vi "ExperimentCode.vi"() -> ()   [LabVIEW 2017]
uses:
  <vilib>/Instr/_visa.llb/VISA Configure Serial Port (Instr).vi
  <vilib>/express/express shared/transition.llb/Dynamic To Waveform Array.vi
  <vilib>/express/express signal manip/GetorSetDDTAttributes/Set DDT Attributes/SetT0.vi
  <vilib>/express/express shared/transition.llb/Waveform Array To Dynamic.vi
  <vilib>/express/express signal manip/GetorSetDDTAttributes/Set DDT Attributes/Set DDT Properties.xnode
  <vilib>/Analysis/NI_AALPro.lvlib
panel:
  in  "Yaw Moment Intercept":dbl
  in  "Yaw Moment Slope":dbl
  in  "Lift Force Intercept":dbl
  in  "Lift Force Slope":dbl
  in  "Drag Force Intercept":dbl
  in  "Drag Force Slope":dbl
  in  "Tab Control":enum32{"Setup ", "Experiment Controls", "Debug"}(tab)=enum."Experiment Controls"
  in  "Max Torque":dbl=21.3
  in  "Servo 1 Zero Offset":dbl
  in  "Servo 2 Zero Offset":dbl
  in  "Servo 3 Zero Offset":dbl
  in  "Servo 4 Zero Offset":dbl
  in  "Servo 5 Zero Offset":dbl
  in  "Servo 5 Torque Intercept":dbl=-52.5
  in  "Servo 5 Torque Slope":dbl=0.0021
  in  "Servo 5 Position Intercept":dbl=-125.0
  in  "Servo 5 Position Slope":dbl=0.007
  in  "Servo 4 Torque Intercept":dbl=-52.5
  in  "Servo 4 Torque Slope":dbl=0.0021
  in  "Servo 4 Position Intercept":dbl=-125.0
  in  "Servo 4 Position Slope":dbl=0.007
  in  "Servo 3 Torque Intercept":dbl=-52.5
  in  "Servo 3 Torque Slope":dbl=0.0021
  in  "Servo 3 Position Intercept":dbl=-125.0
  in  "Servo 3 Position Slope":dbl=0.007
  in  "Servo 2 Torque Intercept":dbl=-52.5
  in  "Servo 2 Torque Slope":dbl=0.0021
  in  "Servo 2 Position Intercept":dbl=-125.0
  in  "Servo 2 Position Slope":dbl=0.007
  in  "Servo 1 Torque Intercept":dbl=-52.5
  in  "Servo 1 Torque Slope":dbl=0.0021
  in  "Servo 1 Position Intercept":dbl=-125.0
  in  "Servo 1 Position Slope":dbl=0.007
  in  "Plot Last x Seconds":dbl=5.0
  in  "COM Port":refnum<visa-resource-name>
  in  "Buad Rate":i32(ring)=115200 items=["2400"=2400, "4800"=4800, "9600"=9600, "14400"=14400, "19200"=19200, "28800"=28800, "38400"=38400, "57600"=57600, "115200"=115200]
  in  "Lowest Servo Angle":dbl=15.0
  in  "Highest Servo Angle":dbl=155.0
  out "Lift FFT":cluster{"timeout (s)":dbl, dbl, dbl[]}(graph)
  out "Maximum Torque Exceeded":bool
  in  "Amplitude (deg)":dbl=3.0
  in  "Save":bool
  in  "Stop VI":bool
  in  "Sample Frequency":dbl=10000.0 step=50.0
  out "Servo Torque":cluster{" Time Offset":dbl, dbl, dbl[][]}(graph)
  in  "Amplitude":dbl=4.0
  in  "Length of Segments":dbl=10.0
  in  "Number of Servos":dbl=5.0
  in  "Number of Waves":dbl=1.0
  in  "Wave Exponential":dbl=2.0
  in  "Frequency":dbl=1.0
  in  "Wave Form":u16(ring) items=["Sine", "Exponentional Sine", "Second Mode Bending", "Flat Plate"]
  in  "Wind Up Waveform":bool
  in  "Mode 1 Amplitude":dbl=0.1 step=0.1
  in  "Mode 2 Amplitude":dbl=0.2 step=0.1
  in  "Mode 1 Phase":dbl step=0.1
  in  "Mode 2 Phase":dbl=0.8499 step=0.1
  in  "Wind Down Waveform":bool
  in  "Wind Down Time":i32=5
  out "Waveform":cluster{"X Nodes":dbl[], "Y Nodes":dbl[]}[](graph)
  in  "Servo Input":bool
  in  "Send To Waveform to MBE":bool
  in  "Servo 5 Input":dbl=90.0
  in  "Servo 4 Input":dbl=90.0
  in  "Servo 3 Input":dbl=90.0
  in  "Servo 2 Input":dbl=90.0
  in  "Servo 1 Input":dbl=90.0
  out "Force and Torque Data":cluster{i32, dbl, dbl[][]}(graph)
  out "Minimum or Maximum Angle Exceeded":bool
  in  "Filename":path=path "test.tdms"
  in  "Comment":string
  out "Output Angles":dbl[](array[numeric])
  out "Input Angles":dbl[](array[numeric])
  out "Pos5 number":dbl
  out "Pos4 number":dbl
  out "Pos3 number":dbl
  out "Pos2 number":dbl
  out "Pos1 number":dbl
  out "Torq1 number":dbl
  out "Torq2 number":dbl
  out "Torq3 number":dbl
  out "Torq4 number":dbl
  out "Torq5 number":dbl
  out "Servo 1 Position":cluster{i32, dbl, dbl[][]}(graph)
  out "Servo 2 Position":cluster{i32, dbl, dbl[][]}(graph)
  out "Servo 3 Position":cluster{i32, dbl, dbl[][]}(graph)
  out "Servo 4 Position":cluster{i32, dbl, dbl[][]}(graph)
  out "Servo 5 Position":cluster{i32, dbl, dbl[][]}(graph)
  out "Sent to Arduino":string
  out "Bytes at port":cluster{i32, dbl, dbl[]}(graph)
  out "Read Buffer":string
  # "deg"
  # "deg"
  # "deg"
  # "deg"
  # "deg"
  # "Waveform"
  # "Manual"
  # "cm"
  # "cm"
  # "Hz"
  # "Off"
  # "On"
  # "rad"
  # "rad"
  # "Off"
  # "On"
  # "Hz"
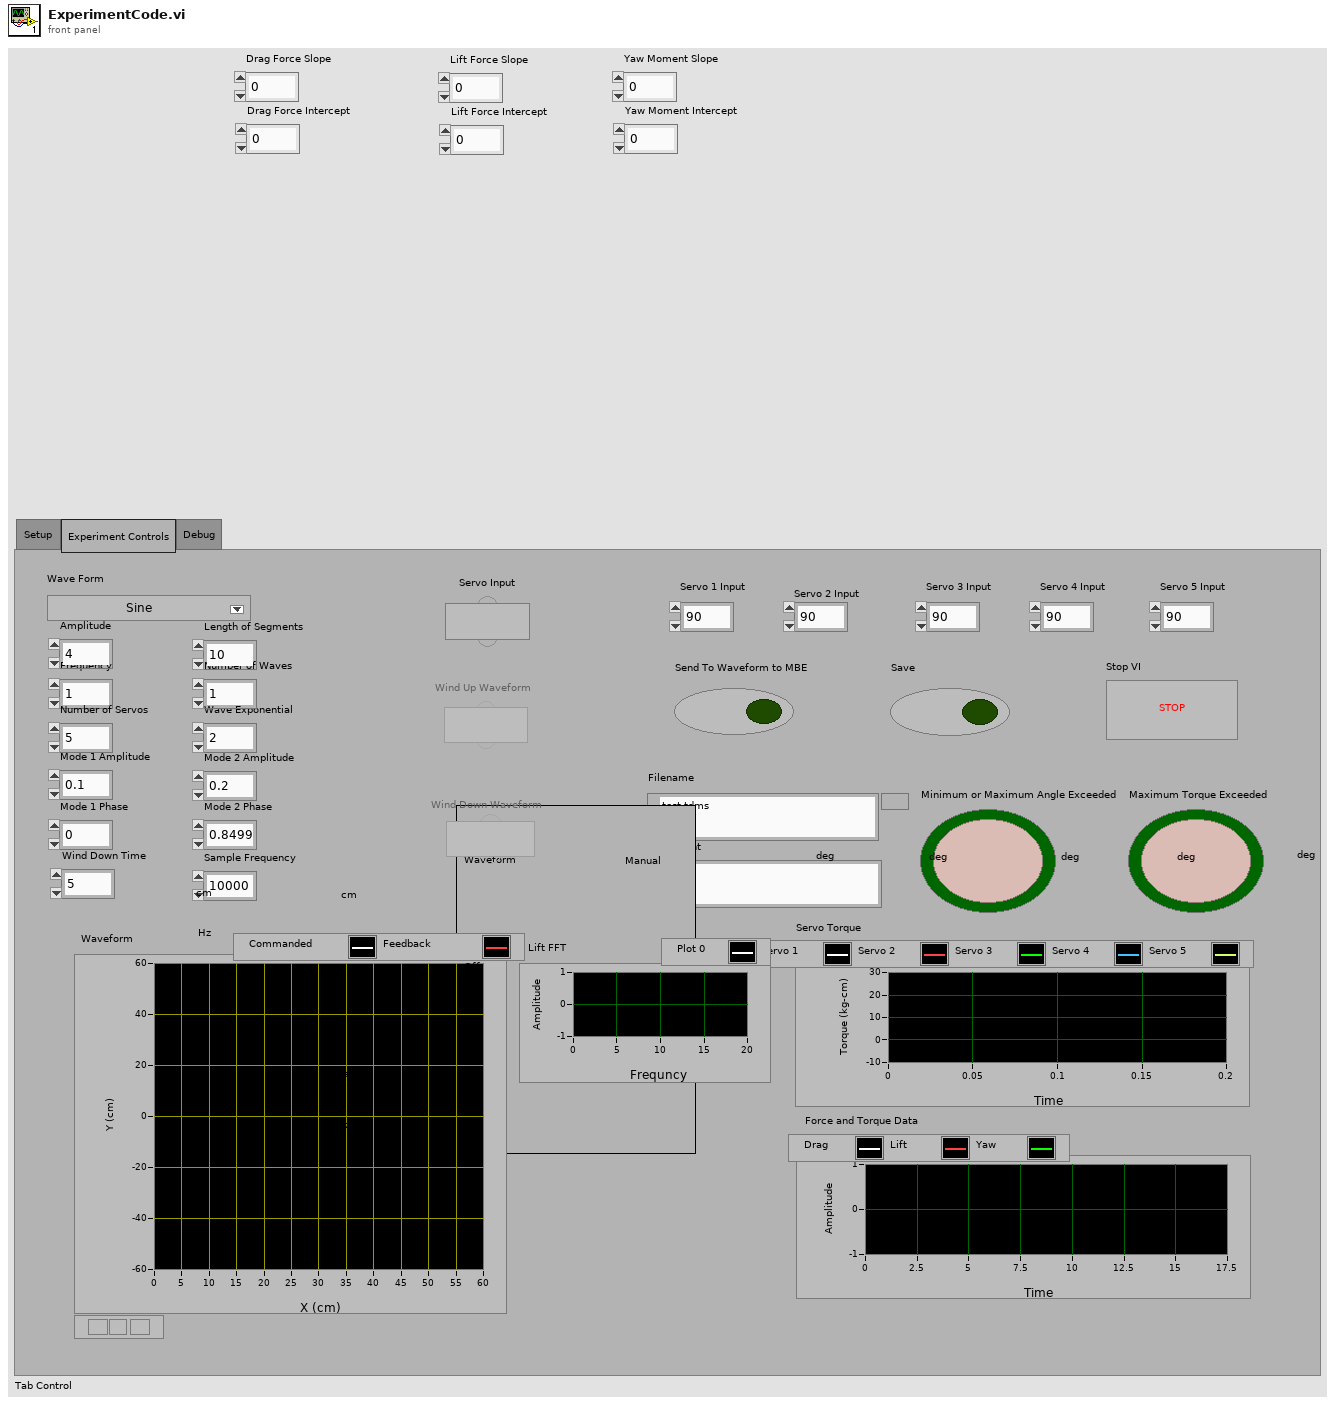
[diagram p1: front panel]
types:
  T1 = enum8{"Enabled", "Disabled", "Disabled and Grayed Out"}
  T2 = cluster{"Amplitude (deg)":dbl, "Amplitude":dbl, "Frequency":dbl, "Number of Waves":dbl, "Length of Segments":dbl, "Wave Exponential":dbl, "Number of Servos":dbl, "Mode 1 Amplitude":dbl, "Mode 2 Amplitude":dbl, "Mode 1 Phase":dbl, "Mode 2 Phase":dbl}
  T3 = cluster{"timeout (s)":dbl, "df":dbl, "Amp Spectrum Mag (Vrms)":dbl[]}
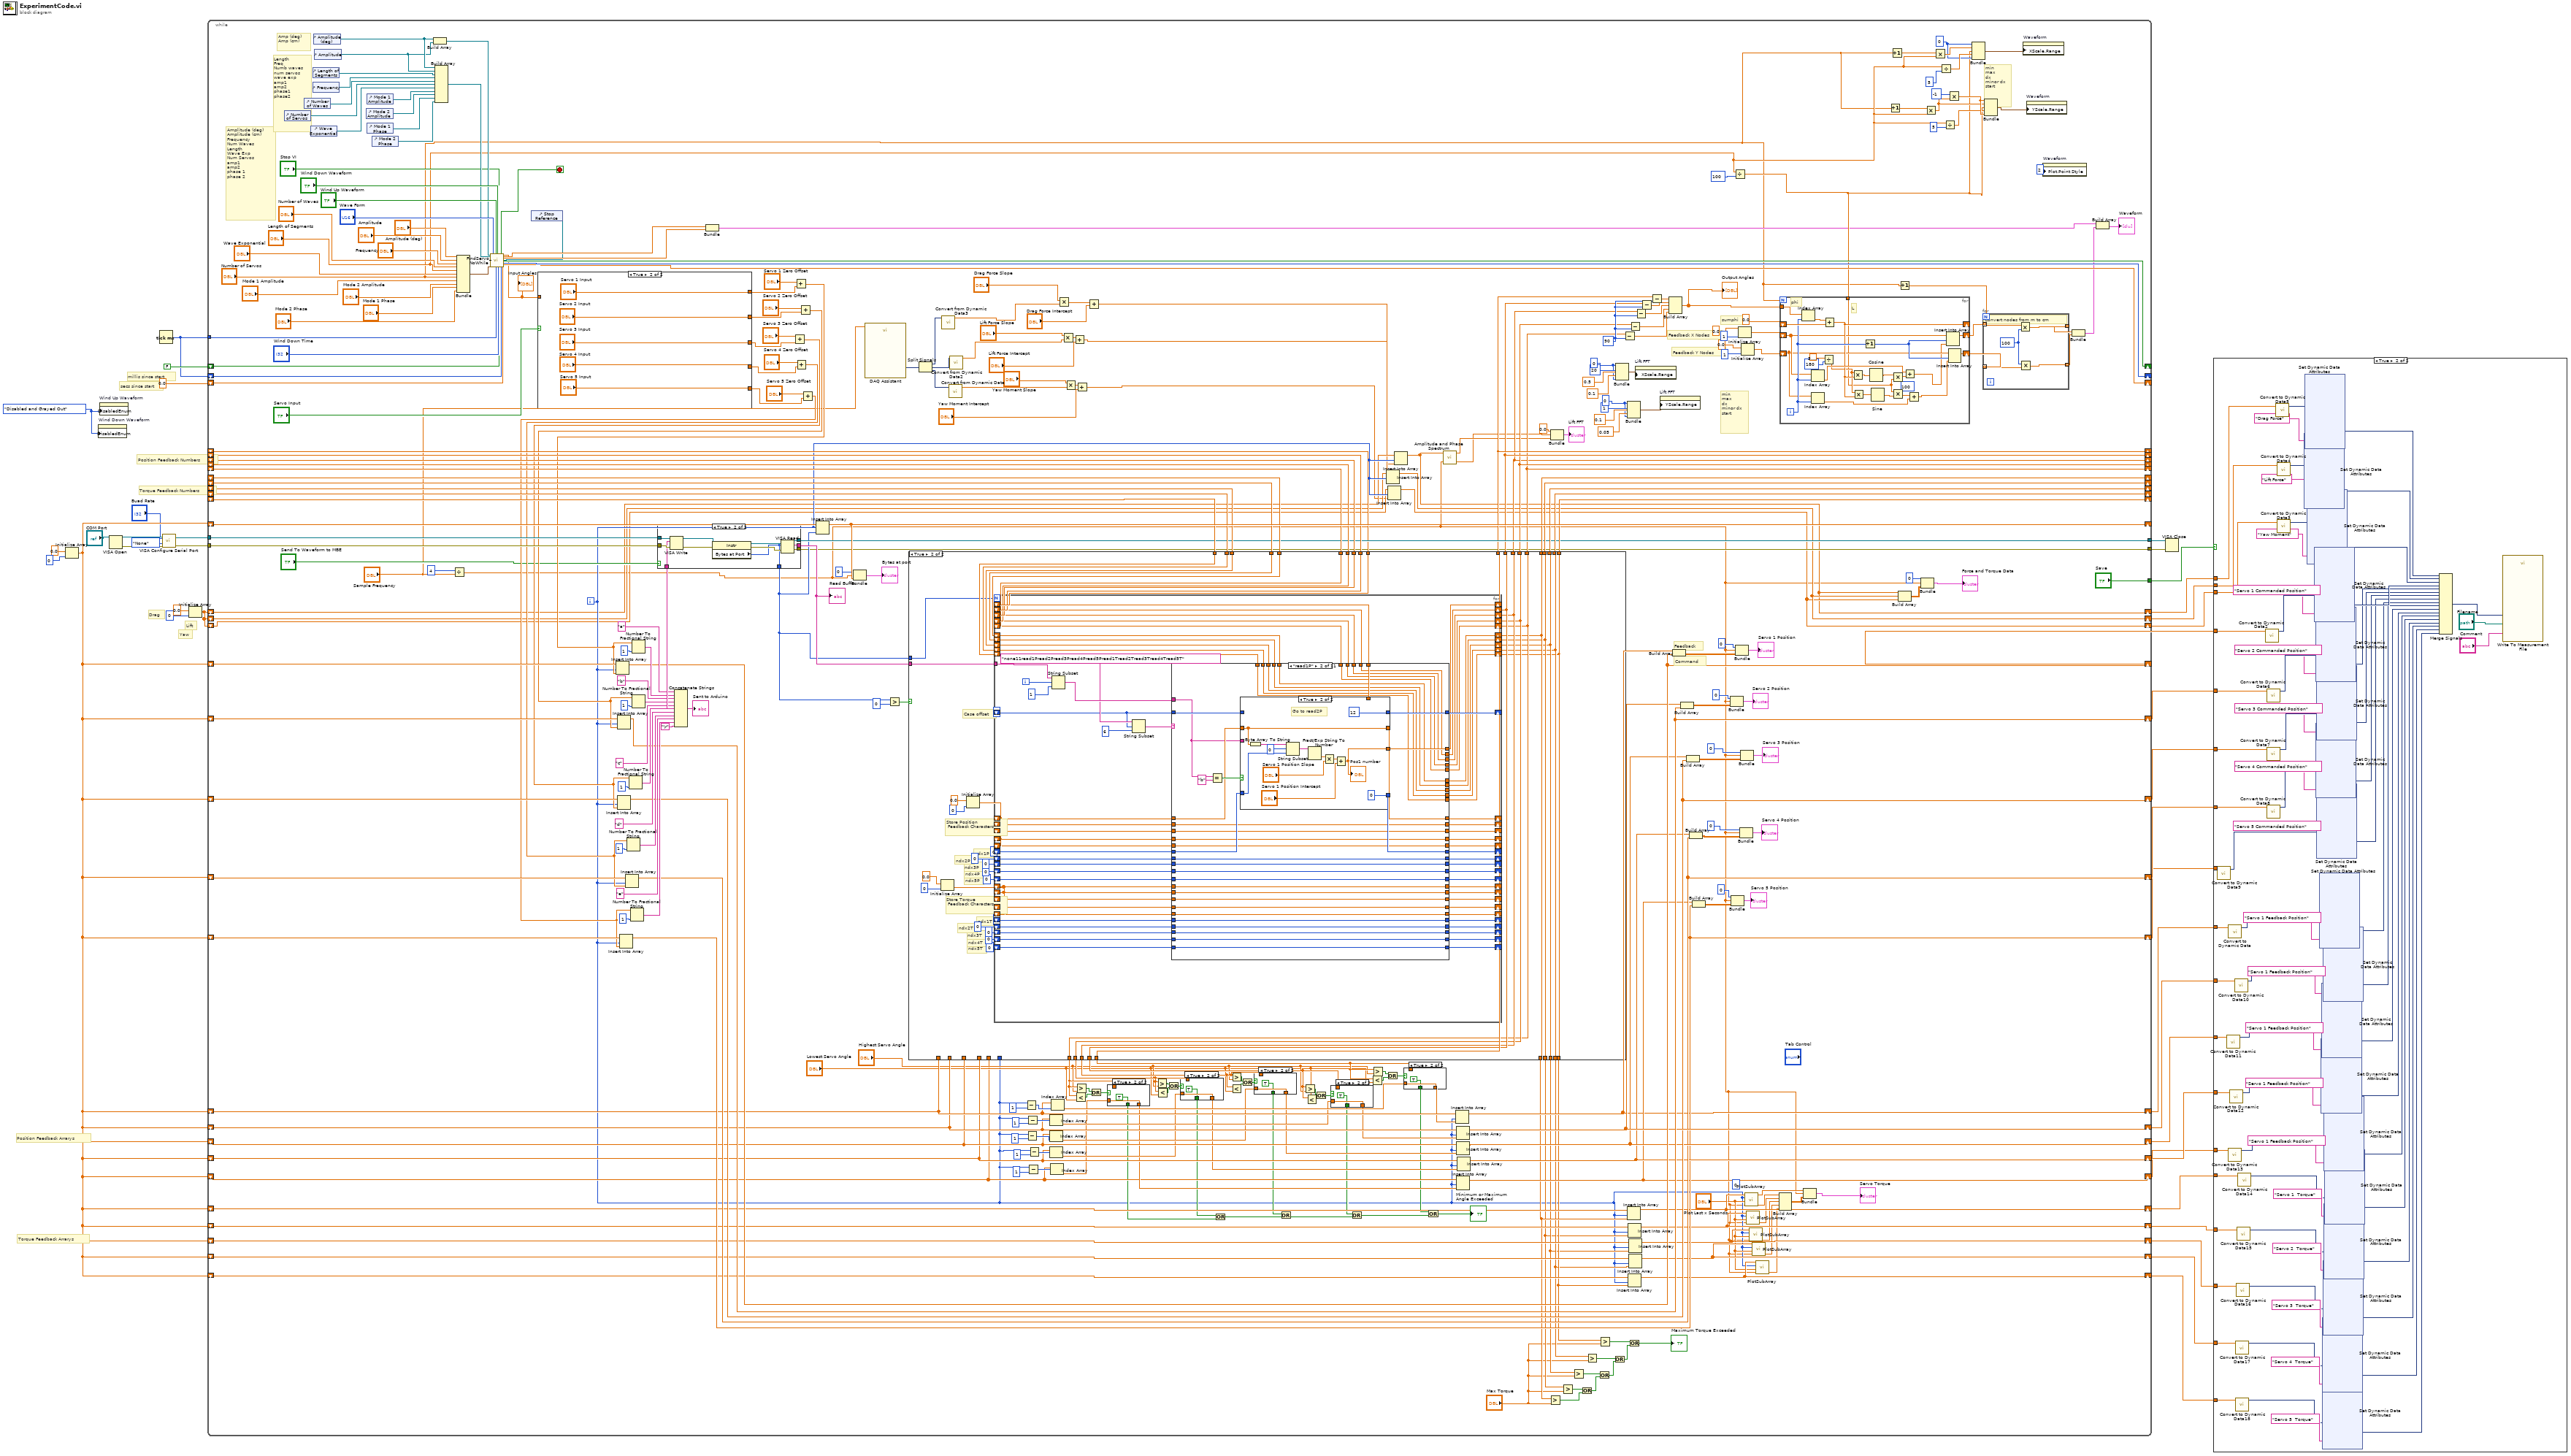
[diagram p0: block diagram]
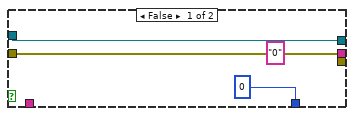
[diagram p3: hidden frame]
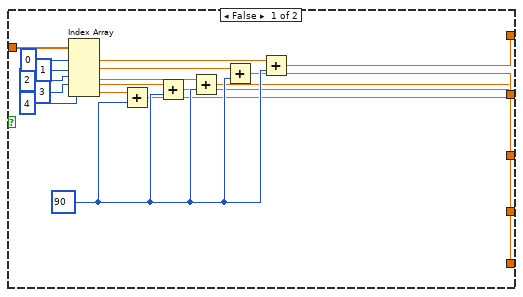
[diagram p4: hidden frame]
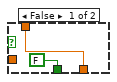
[diagram p5: hidden frame]
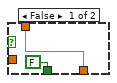
[diagram p6: hidden frame]
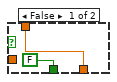
[diagram p7: hidden frame]
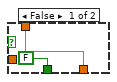
[diagram p8: hidden frame]
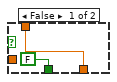
[diagram p9: hidden frame]
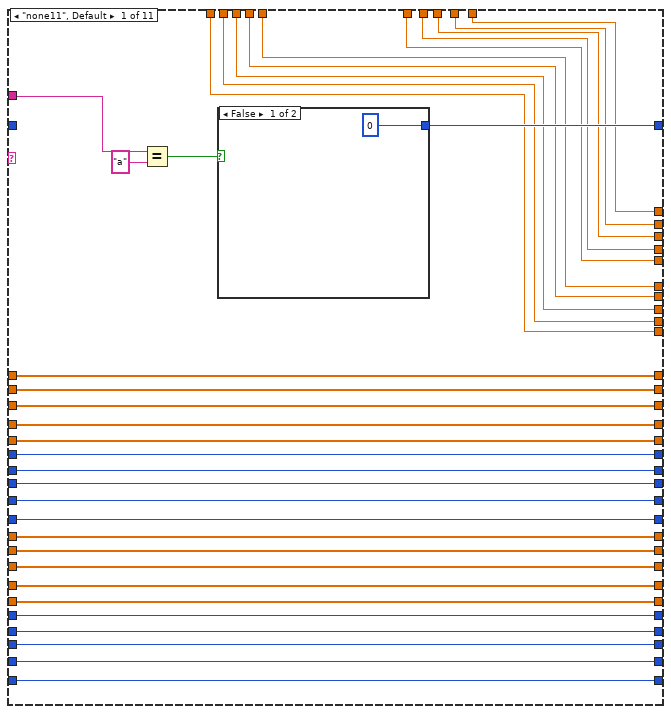
[diagram p11: hidden frame]
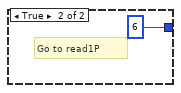
[diagram p12: hidden frame]
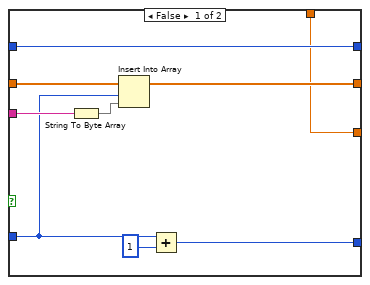
[diagram p13: hidden frame]
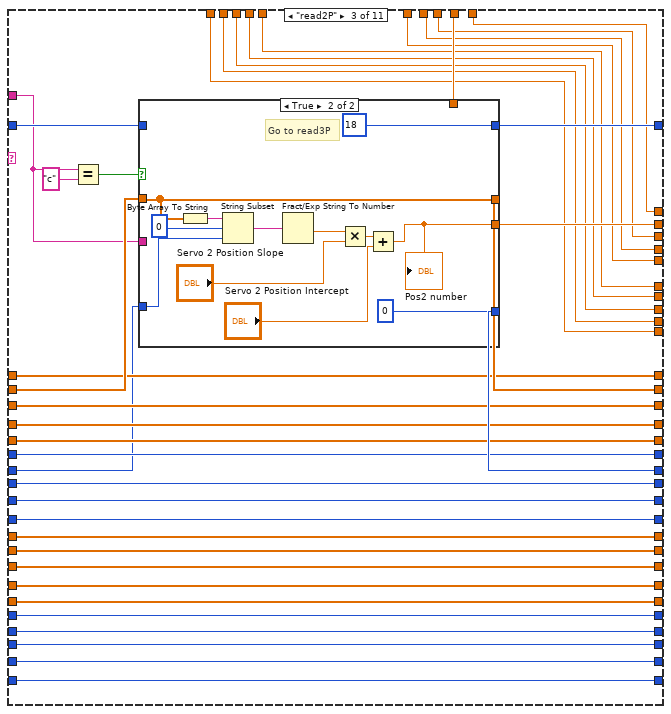
[diagram p14: hidden frame]
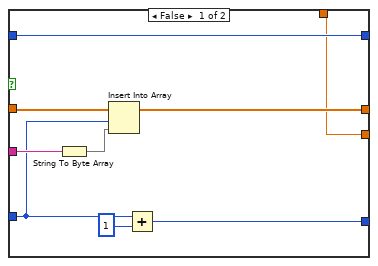
[diagram p15: hidden frame]
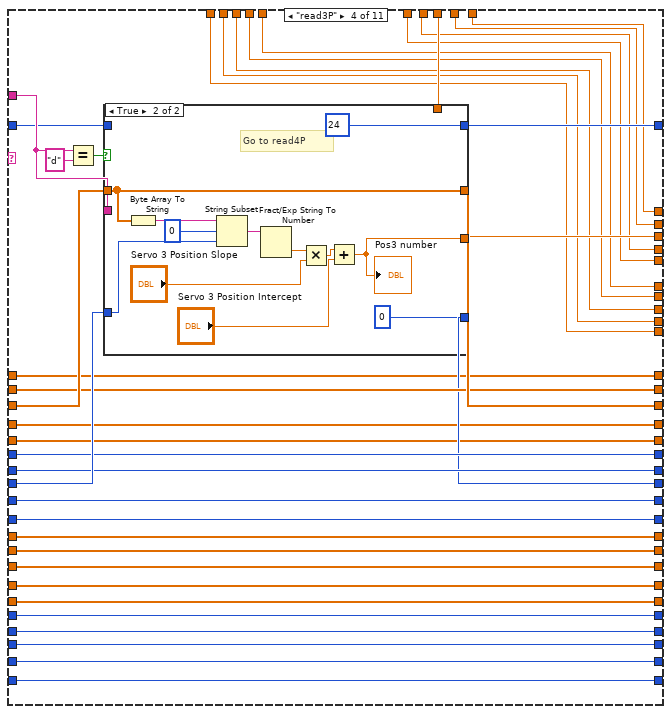
[diagram p16: hidden frame]
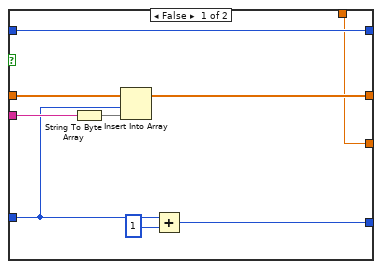
[diagram p17: hidden frame]
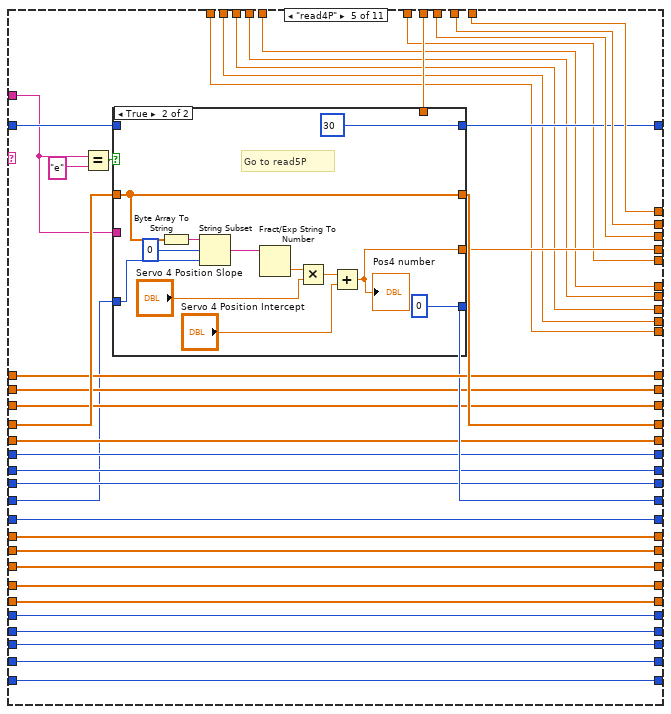
[diagram p18: hidden frame]
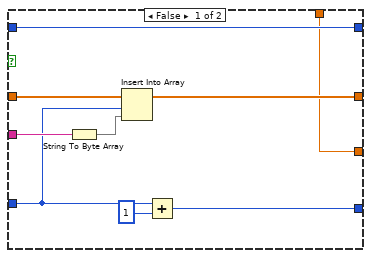
[diagram p19: hidden frame]
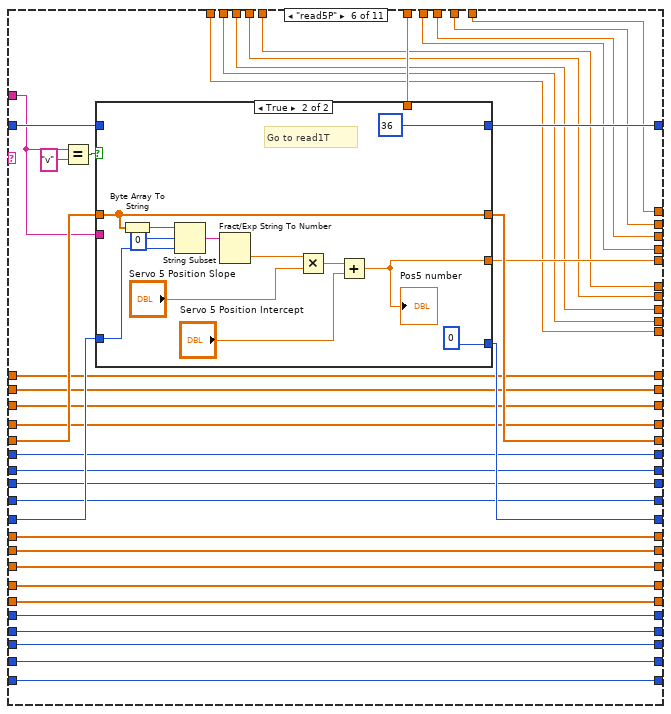
[diagram p20: hidden frame]
diagram:
  w17 = T1."Disabled and Grayed Out" ("Disabled")
  # "Yaw"
  # "Lift"
  # "secs since start"
  # "millis since start"
  # "Drag"
  # "Torque Feedback Numbers"
  # "Position Feedback Numbers"
  # "Torque Feedback Arrarys"
  # "Position Feedback Arrarys"
  n1 = Initialize Array(0.0 ("element"), 0 ("dimension size")) -> (w35:dbl[])
  n2 = property on="Wind Down Waveform" class="Bool (strict)"("DisabledEnum"=w17) -> ()  [unwired: 2 in, 2 out]
  n3 = property on="Wind Up Waveform" class="Bool (strict)"("DisabledEnum"=w17) -> ()  [unwired: 2 in, 2 out]
  n4 = VISA Open(VISA resource name="COM Port") -> (VISA resource name=w34:refnum<visa-resource-name>, error out=w32:errorcluster)  [unwired: 4 in]
  n5 = Tick Count (ms)() -> (millisecond timer value=w26:u32)
  n6 = call-poly "VISA Configure Serial Port"("VISA resource name"=w34, "baud rate (9600)"="Buad Rate", "parity (0:none)"=enum16{"None", "Odd", "Even", "Mark", "Space"}."None", "error in (no error)"=w32) -> ("VISA resource name out"=w30:refnum<visa-resource-name>, "error out"=w31:errorcluster)  [unwired: 10 in]
  n7 = Initialize Array(0.0 ("element"), 0 ("dimension size")) -> (w18:dbl[])
  n8 = while {
    shift-right: [w350] -> _
    shift-left: w35 -> [w351]
    shift-right: [w313] -> w24
    shift-left: w35 -> [w328]
    shift-right: [w310] -> w13
    shift-left: w35 -> [w327]
    shift-right: [w307] -> w12
    shift-left: w35 -> [w326]
    shift-right: [w304] -> w11
    shift-left: w35 -> [w325]
    shift-right: [w301] -> w10
    shift-left: w35 -> [w324]
    shift-right: [w147] -> w20
    shift-left: w35 -> [w274]
    shift-right: [w309] -> w9
    shift-left: w35 -> [w266]
    shift-right: [w306] -> w8
    shift-left: w35 -> [w263]
    shift-right: [w303] -> w7
    shift-left: w35 -> [w260]
    shift-right: [w300] -> w6
    shift-left: w35 -> [w230]
    shift-right: [w116] -> _
    shift-left: _ -> [w277]
    shift-right: [w115] -> _
    shift-left: _ -> [w296]
    shift-right: [w112] -> _
    shift-left: _ -> [w299]
    shift-right: [w114] -> _
    shift-left: _ -> [w298]
    shift-right: [w113] -> _
    shift-left: _ -> [w297]
    shift-right: [w290] -> _
    shift-left: _ -> [w291]
    shift-right: [w289] -> _
    shift-left: _ -> [w292]
    shift-right: [w288] -> _
    shift-left: _ -> [w293]
    shift-right: [w287] -> _
    shift-left: _ -> [w294]
    shift-right: [w286] -> _
    shift-left: _ -> [w295]
    shift-right: [w160] -> w5
    shift-left: w35 -> [w285]
    shift-right: [w158] -> w4
    shift-left: w35 -> [w284]
    shift-right: [w157] -> w3
    shift-left: w35 -> [w283]
    shift-right: [w156] -> w2
    shift-left: w35 -> [w282]
    shift-right: [w159] -> w1
    shift-left: w35 -> [w281]
    tunnel: w31 -> [w229]
    shift-right: [w74] -> w16
    shift-left: w18 -> [w79]
    tunnel: w26 -> [w224]
    shift-right: [w220] -> _
    shift-left: FALSE -> [w214]
    shift-right: [w219] -> _
    shift-left: w26 -> [w222]
    shift-right: [w218] -> _
    shift-left: 0.0 ("S since stop Shift Out") -> [w221]
    tunnel: ["Save"] -> w23
    tunnel: w30 -> [w228]
    tunnel: [w278] -> w22
    tunnel: [w84] -> w21
    shift-right: [w76] -> w15
    shift-left: w18 -> [w78]
    shift-right: [w75] -> w14
    shift-left: w18 -> [w77]
    i -> [w80]
    stop <- w170 stop-if-true
    w61 = 0
    w65 = 0
    w101 = 0
    w117 = 90
    (unwired) 0
    # "min\nmax\ndx\nminor dx\nstart"
    # "min\nmax\ndx\nminor dx\nstart"
    # "Feedback Y Nodes"
    # "Feedback X Nodes"
    # "sumphi"
    # "Command"
    # "Feedback"
    # "Amplitude (deg)\nAmplitude (cm)\nFrequency\nNum Waves\nLength\nWave Exp\nNum Servos\namp1\namp2\nphase 1\nphase 2"
    # "Amp (deg)\nAmp (cm)"
    # "Length\nFreq\nNumb waves\nnum servos\nwave exp\namp1\namp2\nphase1\nphase2"
    n9 = control-ref of="Number of Servos"() -> (w193:refnum<vi>)
    n10 = control-ref of="Number of Waves"() -> (w194:refnum<vi>)
    n11 = control-ref of="Wave Exponential"() -> (w192:refnum<vi>)
    n12 = control-ref of="Length of Segments"() -> (w196:refnum<vi>)
    n13 = control-ref of="Frequency"() -> (w195:refnum<vi>)
    n14 = control-ref of="Amplitude (deg)"() -> (w175:refnum<vi>)
    n15 = control-ref of="Amplitude"() -> (w174:refnum<vi>)
    n16 = control-ref of="Mode 2 Amplitude"() -> (w190:refnum<vi>)
    n17 = control-ref of="Mode 1 Amplitude"() -> (w191:refnum<vi>)
    n18 = control-ref of="Mode 1 Phase"() -> (w189:refnum<vi>)
    n19 = control-ref of="Mode 2 Phase"() -> (w188:refnum<vi>)
    n20 = Build Array(w175, w174) -> (w177:refnum<vi>[])
    n21 = Build Array(w175, w174, w196, w195, w194, w193, w192, w191, w190, w189, w188) -> (w176:refnum<vi>[])
    n22 = Divide(x=4, y="Sample Frequency") -> (x/y=w39:dbl)
    n23 = Bundle("Amplitude (deg)"="Amplitude (deg)", "Amplitude"="Amplitude", "Frequency"="Frequency", "Number of Waves"="Number of Waves", "Length of Segments"="Length of Segments", "Wave Exponential"="Wave Exponential", "Number of Servos"="Number of Servos", "Mode 1 Amplitude"="Mode 1 Amplitude", "Mode 2 Amplitude"="Mode 2 Amplitude", "Mode 1 Phase"="Mode 1 Phase", "Mode 2 Phase"="Mode 2 Phase") -> (w178:T2)  [unwired: 1 in]
    n24 = control-ref of="Stop Reference"() -> (w213:refnum<vi>)
    n25 = call "FindServo_NoWhile.vi"("Amplitude Reference Array"=w177, "Parameter Reference Arrary"=w176, "Parameter Cluster"=w178, "Wave Form"="Wave Form", "Wind Up"="Wind Up Waveform", "Start Time (Tick Count-millis)"=w224, "Wind Down"="Wind Down Waveform", "Wind Down Time"="Wind Down Time", "Stop In"="Stop VI", "Stop Pressed Shift In (False)"=w214, "Ms Since Stop Shift In (Start Time)"=w222, "Stop In Reference"=w213, "S since stop Shift In"=w221) -> ("Stop Out"=w170:bool, "phi"=w85:dbl[], "X Nodes"=w217:dbl[], "Y Nodes"=w216:dbl[], "Stop Pressed Shift Out (False)"=w220:bool, "MS Since Stop Shift Out"=w219:u32, "S since stop Shift Out"=w218:dbl)  [unwired: 8 in]
    "Input Angles" <- w85
    n26 = case shown="True" "Servo Input" {
      tunnel: [w400 "Servo 1 Input"] -> w207
      tunnel: [w399 "Servo 2 Input"] -> w206
      tunnel: [w398 "Servo 3 Input"] -> w205
      tunnel: [w397 "Servo 4 Input"] -> w204
      tunnel: [w396 "Servo 5 Input"] -> w203
      tunnel: w85 -> [w412 _]
      frame False {
        w401 = 90
        n27 = Index Array(array=w412, index #1=0, index #2=1, index #3=2, index #4=3, index #5=4) -> (element #1=w406:dbl, element #2=w405:dbl, element #3=w404:dbl, element #4=w403:dbl, element #5=w402:dbl)
        n28 = Add(x=w402, y=w401) -> (x+y=w396:dbl)
        n29 = Add(x=w403, y=w401) -> (x+y=w397:dbl)
        n30 = Add(x=w404, y=w401) -> (x+y=w398:dbl)
        n31 = Add(x=w405, y=w401) -> (x+y=w399:dbl)
        n32 = Add(x=w406, y=w401) -> (x+y=w400:dbl)
      }
      frame True {
      }
    }
    n33 = Bundle("X Nodes"=w217, "Y Nodes"=w216) -> (w96:cluster{"X Nodes":dbl[], "Y Nodes":dbl[]})  [unwired: 1 in]
    n34 = Add(x="Servo 3 Zero Offset", y=w205) -> (x+y=w200:dbl)
    n35 = Insert Into Array(array=w326, index=w80, new element=w200) -> (w307:dbl[])
    n36 = Number To Fractional String(number=w200, precision (6)=1) -> (F-format string=w346:string)  [unwired: 2 in]
    n37 = Add(x="Servo 1 Zero Offset", y=w207) -> (x+y=w198:dbl)
    n38 = Insert Into Array(array=w328, index=w80, new element=w198) -> (w313:dbl[])
    n39 = Number To Fractional String(number=w198, precision (6)=1) -> (F-format string=w348:string)  [unwired: 2 in]
    n40 = Add(x="Servo 4 Zero Offset", y=w204) -> (x+y=w201:dbl)
    n41 = Insert Into Array(array=w325, index=w80, new element=w201) -> (w304:dbl[])
    n42 = Number To Fractional String(number=w201, precision (6)=1) -> (F-format string=w339:string)  [unwired: 2 in]
    n43 = Add(x="Servo 2 Zero Offset", y=w206) -> (x+y=w199:dbl)
    n44 = Insert Into Array(array=w327, index=w80, new element=w199) -> (w310:dbl[])
    n45 = Number To Fractional String(number=w199, precision (6)=1) -> (F-format string=w347:string)  [unwired: 2 in]
    n46 = Add(x="Servo 5 Zero Offset", y=w203) -> (x+y=w202:dbl)
    n47 = Insert Into Array(array=w324, index=w80, new element=w202) -> (w301:dbl[])
    n48 = Number To Fractional String(number=w202, precision (6)=1) -> (F-format string=w338:string)  [unwired: 2 in]
    n49 = Concatenate Strings("a", w348, "b", w347, "c", w346, "d", w339, "e", w338, "\r") -> (w349:string)
    "Sent to Arduino" <- w349
    n50 = case shown="True" "Send To Waveform to MBE" {
      tunnel: w349 -> [_ w385]
      tunnel: ["0" w395] -> w335
      tunnel: [w383 w394] -> w84
      tunnel: [w384 w393] -> w278
      tunnel: [0 w388] -> w173
      tunnel: w229 -> [w383 w387]
      tunnel: w228 -> [w384 w386]
      frame False {
      }
      frame True {
        n51 = VISA Write(VISA resource name=w386, write buffer=w385, error in (no error)=w387) -> (VISA resource name out=w392:refnum<visa-resource-name>, error out=w389:errorcluster)  [unwired: 1 out]
        n52 = property class="Instr"(reference=w392, error in=w389) -> (reference out=w391:refnum<visa-resource-name>, error out=w390:errorcluster, "Bytes at Port"=w388:u32)
        n53 = VISA Read(VISA resource name=w391, byte count=w388, error in (no error)=w390) -> (VISA resource name out=w393:refnum<visa-resource-name>, read buffer=w395:string, error out=w394:errorcluster)  [unwired: 1 out]
      }
    }
    "Read Buffer" <- w335
    n54 = Insert Into Array(array=w351, index=w80, new element=w173) -> (w350:dbl[])
    n55 = Bundle(0, w39, w350) -> (→"Bytes at port":cluster{i32, dbl, dbl[]})  [unwired: 1 in]
    n56 = call "DAQ Assistant"("rate"="Sample Frequency") -> ("data"=w59:dynamicdata)  [unwired: 16 in, 2 out]
    n57 = Greater?(x=w173, y=0) -> (0:w280:bool)
    n58 = case shown="True" w280 {
      tunnel: w173 -> [_ w448]
      tunnel: w335 -> [_ w486]
      tunnel: [w447 w460] -> w269
      tunnel: w80 -> [_ _]
      tunnel: w274 -> [_ _]
      tunnel: [w446 w459] -> w251
      tunnel: [w445 w458] -> w245
      tunnel: [w444 w457] -> w239
      tunnel: [w443 w456] -> w235
      tunnel: w266 -> [_ _]
      tunnel: w263 -> [_ _]
      tunnel: w260 -> [_ _]
      tunnel: w230 -> [_ _]
      tunnel: w277 -> [w447 w477]
      tunnel: w296 -> [w446 w476]
      tunnel: w299 -> [w445 w475]
      tunnel: w298 -> [w444 w474]
      tunnel: w297 -> [w443 w473]
      tunnel: [w447 w460] -> w116
      tunnel: [w446 w459] -> w115
      tunnel: [w445 w458] -> w112
      tunnel: [w444 w457] -> w114
      tunnel: [w443 w456] -> w113
      tunnel: w295 -> [w438 w450]
      tunnel: w294 -> [w439 w452]
      tunnel: w293 -> [w440 w472]
      tunnel: w292 -> [w441 w471]
      tunnel: w291 -> [w442 w470]
      tunnel: [w442 w455] -> w290
      tunnel: [w441 w454] -> w289
      tunnel: [w440 w453] -> w288
      tunnel: [w439 w451] -> w287
      tunnel: [w438 w449] -> w286
      tunnel: [w442 w455] -> w145
      tunnel: [w441 w454] -> w141
      tunnel: [w440 w453] -> w142
      tunnel: [w439 w451] -> w143
      tunnel: [w438 w449] -> w144
      frame False {
      }
      frame True {
        # "Store Torque\n Feedback Characters"
        # "ndx5T"
        # "ndx4T"
        # "ndx3T"
        # "ndx2T"
        # "ndx1T"
        # "Store Position\n Feedback Characters"
        # "ndx5P"
        # "ndx4P"
        # "ndx3P"
        # "ndx2P"
        # "ndx1P"
        # "Case offset"
        n59 = Initialize Array(0.0 ("element"), 0 ("dimension size")) -> (w467:dbl[])
        n60 = Initialize Array(0.0 ("element"), 0 ("dimension size")) -> (w480:dbl[])
        n61 = for {
          N: w448 -> [_]
          tunnel: w486 -> [w554]
          shift-right: [w552] -> _
          shift-left: 1 -> [w497]
          shift-right: [w551] -> _
          shift-left: 0 -> [w550]
          shift-right: [w548] -> _
          shift-left: w480 -> [w549]
          shift-right: [w546] -> _
          shift-left: w480 -> [w547]
          shift-right: [w542] -> _
          shift-left: 0 -> [w545]
          shift-right: [w543] -> _
          shift-left: 0 -> [w544]
          shift-right: [w540] -> _
          shift-left: w480 -> [w541]
          shift-right: [w532] -> _
          shift-left: w480 -> [w539]
          shift-right: [w533] -> _
          shift-left: w480 -> [w538]
          shift-right: [w536] -> _
          shift-left: 0 -> [w537]
          shift-right: [w534] -> _
          shift-left: 0 -> [w535]
          shift-right: [w519] -> _
          shift-left: w467 -> [w520]
          shift-right: [w518] -> _
          shift-left: w467 -> [w517]
          shift-right: [w516] -> _
          shift-left: w467 -> [w515]
          shift-right: [w514] -> _
          shift-left: w467 -> [w513]
          shift-right: [w512] -> _
          shift-left: w467 -> [w511]
          shift-right: [w510] -> _
          shift-left: 0 -> [w509]
          shift-right: [w508] -> _
          shift-left: 0 -> [w507]
          shift-right: [w506] -> _
          shift-left: 0 -> [w505]
          shift-right: [w503] -> _
          shift-left: 0 -> [w504]
          shift-right: [w502] -> _
          shift-left: 0 -> [w501]
          shift-right: [w496] -> w460
          shift-left: w477 -> [w527]
          shift-right: [w495] -> w459
          shift-left: w476 -> [w531]
          shift-right: [w494] -> w458
          shift-left: w475 -> [w530]
          shift-right: [w493] -> w457
          shift-left: w474 -> [w529]
          shift-right: [w492] -> w456
          shift-left: w473 -> [w528]
          shift-right: [w491] -> w455
          shift-left: w470 -> [w521]
          shift-right: [w490] -> w454
          shift-left: w471 -> [w522]
          shift-right: [w489] -> w453
          shift-left: w472 -> [w523]
          shift-right: [w488] -> w451
          shift-left: w452 -> [w524]
          shift-right: [w487] -> w449
          shift-left: w450 -> [w525]
          i -> [w498]
          n62 = String Subset(string=w554, offset (0)=w498, length (rest)=1 ("length (rest)")) -> (substring=w526:string)
          n63 = String Subset(string="none11read1Pread2Pread3Pread4Pread5Pread1Tread2Tread3Tread4Tread5T", offset (0)=w497, length (rest)=6 ("length (rest)")) -> (substring=w500:string)
          n64 = case shown="\"read1P\"" w500 {
            tunnel: w526 -> [w589 w623 w679 w733 w800 w859 w920 w979 w1038 w1097 w1156]
            tunnel: [w586 w626 w681 w740 w786 w862 w923 w982 w1041 w1100 w1159] -> w552
            tunnel: [w585 w621 w683 w745 w798 w852 w915 w974 w1033 w1092 w1151] -> w551
            tunnel: w550 -> [w585 w622 w683 w745 w798 w852 w915 w974 w1033 w1092 w1151]
            tunnel: w549 -> [w582 w624 w678 w728 w804 w856 w919 w978 w1037 w1096 w1155]
            tunnel: [w582 w627 w678 w728 w804 w856 w919 w978 w1037 w1096 w1155] -> w548
            tunnel: w547 -> [w583 w620 w688 w741 w796 w855 w918 w977 w1036 w1095 w1154]
            tunnel: [w583 w620 w687 w741 w796 w855 w918 w977 w1036 w1095 w1154] -> w546
            tunnel: w545 -> [w584 w616 w666 w744 w797 w851 w914 w973 w1032 w1091 w1150]
            tunnel: [w584 w616 w686 w744 w797 w851 w914 w973 w1032 w1091 w1150] -> w542
            tunnel: w497 -> [_ w625 w682 w725 w801 w861 w922 w981 w1040 w1099 w1158]
            tunnel: w544 -> [w579 w615 w680 w746 w793 w850 w913 w972 w1031 w1090 w1149]
            tunnel: [w579 w615 w680 w737 w793 w850 w913 w972 w1031 w1090 w1149] -> w543
            tunnel: w541 -> [w576 w619 w677 w743 w795 w854 w917 w976 w1035 w1094 w1153]
            tunnel: [w576 w619 w677 w742 w795 w854 w917 w976 w1035 w1094 w1153] -> w540
            tunnel: w539 -> [w577 w618 w676 w736 w806 w853 w916 w975 w1034 w1093 w1152]
            tunnel: w538 -> [w578 w617 w675 w735 w794 w864 w907 w966 w1018 w1077 w1136]
            tunnel: w537 -> [w581 w614 w674 w739 w785 w849 w912 w971 w1030 w1089 w1148]
            tunnel: [w581 w614 w674 w739 w799 w849 w912 w971 w1030 w1089 w1148] -> w536
            tunnel: w535 -> [w580 w613 w673 w738 w792 w858 w904 w955 w1015 w1071 w1133]
            tunnel: [w580 w613 w673 w738 w792 w857 w904 w955 w1015 w1071 w1133] -> w534
            tunnel: [w578 w617 w675 w735 w794 w863 w907 w966 w1018 w1077 w1136] -> w533
            tunnel: [w577 w618 w676 w736 w805 w853 w916 w975 w1034 w1093 w1152] -> w532
            tunnel: [w571 w612 w670 w726 w787 w848 w911 w970 w1029 w1088 w1147] -> w496
            tunnel: w527 -> [w571 w611 w670 w726 w787 w848 w911 w970 w1029 w1088 w1147]
            tunnel: [w575 w610 w672 w732 w791 w843 w908 w967 w1026 w1085 w1144] -> w495
            tunnel: w531 -> [w575 w610 w671 w732 w791 w843 w908 w967 w1026 w1085 w1144]
            tunnel: [w574 w609 w667 w731 w788 w846 w910 w969 w1028 w1087 w1146] -> w494
            tunnel: w530 -> [w574 w609 w667 w730 w788 w846 w910 w969 w1028 w1087 w1146]
            tunnel: [w573 w608 w669 w729 w790 w844 w909 w968 w1027 w1086 w1145] -> w493
            tunnel: w529 -> [w573 w608 w669 w729 w789 w844 w909 w968 w1027 w1086 w1145]
            tunnel: [w572 w607 w668 w727 w769 w847 w900 w950 w1024 w1084 w1143] -> w492
            tunnel: w528 -> [w572 w607 w668 w727 w769 w845 w900 w950 w1024 w1084 w1143]
            tunnel: w525 -> [w566 w602 w661 w720 w780 w838 w888 w946 w1019 w1078 w1142]
            tunnel: w524 -> [w567 w603 w662 w721 w781 w839 w889 w947 w1021 w1083 w1137]
            tunnel: w523 -> [w568 w604 w663 w722 w782 w840 w890 w948 w1025 w1080 w1138]
            tunnel: w522 -> [w569 w605 w664 w723 w783 w841 w891 w952 w1022 w1081 w1139]
            tunnel: w521 -> [w570 w606 w665 w724 w784 w842 w901 w951 w1023 w1082 w1140]
            tunnel: [w570 w606 w665 w724 w784 w842 w899 w951 w1023 w1082 w1140] -> w491
            tunnel: [w569 w605 w664 w723 w783 w841 w891 w949 w1022 w1081 w1139] -> w490
            tunnel: [w568 w604 w663 w722 w782 w840 w890 w948 w1020 w1080 w1138] -> w489
            tunnel: [w567 w603 w662 w721 w781 w839 w889 w947 w1021 w1079 w1137] -> w488
            tunnel: [w566 w602 w661 w720 w780 w838 w888 w946 w1019 w1078 w1141] -> w487
            tunnel: w520 -> [w565 w601 w660 w719 w779 w837 w906 w963 w1012 w1074 w1123]
            tunnel: [w565 w601 w660 w719 w779 w837 w905 w963 w1012 w1074 w1123] -> w519
            tunnel: [w564 w600 w659 w718 w778 w836 w898 w964 w1011 w1073 w1124] -> w518
            tunnel: w517 -> [w564 w600 w659 w718 w778 w836 w898 w965 w1011 w1073 w1124]
            tunnel: [w563 w599 w658 w717 w777 w835 w897 w962 w1016 w1072 w1125] -> w516
            tunnel: w515 -> [w563 w599 w658 w717 w777 w835 w897 w962 w1017 w1072 w1125]
            tunnel: [w562 w598 w657 w716 w776 w834 w896 w961 w1010 w1076 w1126] -> w514
            tunnel: w513 -> [w562 w598 w657 w716 w776 w834 w896 w961 w1010 w1075 w1126]
            tunnel: [w561 w597 w656 w715 w775 w833 w895 w960 w1009 w1067 w1135] -> w512
            tunnel: w511 -> [w561 w597 w656 w715 w775 w833 w895 w960 w1009 w1067 w1134]
            tunnel: [w560 w596 w655 w714 w774 w832 w902 w959 w1008 w1068 w1127] -> w510
            tunnel: w509 -> [w560 w596 w655 w714 w774 w832 w903 w959 w1008 w1068 w1127]
            tunnel: [w559 w595 w654 w713 w773 w831 w894 w954 w1007 w1066 w1128] -> w508
            tunnel: w507 -> [w559 w595 w654 w713 w773 w831 w894 w953 w1007 w1066 w1128]
            tunnel: [w558 w594 w653 w712 w772 w830 w893 w958 w1014 w1065 w1129] -> w506
            tunnel: w505 -> [w558 w594 w653 w712 w772 w830 w893 w958 w1013 w1065 w1129]
            tunnel: w504 -> [w557 w593 w652 w711 w771 w829 w892 w957 w1006 w1069 w1130]
            tunnel: [w557 w593 w652 w711 w771 w829 w892 w957 w1006 w1070 w1130] -> w503
            tunnel: [w556 w592 w651 w710 w770 w828 w887 w956 w1005 w1064 w1132] -> w502
            tunnel: w501 -> [w556 w592 w651 w710 w770 w828 w887 w956 w1005 w1064 w1131]
            frame "none11", Default {
              n65 = Equal?(x=w589, y="a") -> (x = y?=w587:bool)
              n66 = case shown="False" w587 {
                tunnel: [0 6] -> w586
                frame False {
                }
                frame True {
                  # "Go to read1P"
                }
              }
            }
            frame "read1P" {
              n67 = Equal?(x=w623, y="b") -> (x = y?=w628:bool)
              n68 = case shown="True" w628 {
                tunnel: [w638 0] -> w621
                tunnel: w624 -> [w632 w646]
                tunnel: [w636 w646] -> w627
                tunnel: w623 -> [w635 _]
                tunnel: [w633 12] -> w626
                tunnel: w625 -> [w633 _]
                tunnel: w622 -> [w631 w645]
                tunnel: [w630 w643] -> w612
                tunnel: w611 -> [w630 _]
                frame False {
                  n69 = String To Byte Array(string=w635) -> (unsigned byte array=w634:u8[])
                  n70 = Insert Into Array(array=w632, index=w631, new element=w634) -> (w636:dbl[])
                  n71 = Add(x=w631, y=1) -> (x+y=w638:i32)
                }
                frame True {
                  # "Go to read2P"
                  n72 = Byte Array To String(unsigned byte array=w646) -> (string=w647:string)
                  n73 = String Subset(string=w647, offset (0)=0, length (rest)=w645) -> (substring=w644:string)
                  n74 = Fract/Exp String To Number(string=w644) -> (number=w642:dbl)  [unwired: 3 in, 1 out]
                  n75 = Multiply(x=w642, y="Servo 1 Position Slope") -> (x*y=w641:dbl)
                  n76 = Add(x=w641, y="Servo 1 Position Intercept") -> (x+y=w643:dbl)
                  "Pos1 number" <- w643
                }
              }
            }
            frame "read2P" {
              n77 = Equal?(x=w679, y="c") -> (x = y?=w684:bool)
              n78 = case shown="True" w684 {
                tunnel: [w697 0] -> w686
                tunnel: w666 -> [w691 w706]
                tunnel: w688 -> [w695 w704]
                tunnel: [w694 w704] -> w687
                tunnel: w679 -> [w693 _]
                tunnel: [w690 18] -> w681
                tunnel: w682 -> [w690 _]
                tunnel: [w689 w700] -> w672
                tunnel: w671 -> [w689 _]
                frame False {
                  n79 = String To Byte Array(string=w693) -> (unsigned byte array=w692:u8[])
                  n80 = Insert Into Array(array=w695, index=w691, new element=w692) -> (w694:dbl[])
                  n81 = Add(x=w691, y=1) -> (x+y=w697:i32)
                }
                frame True {
                  # "Go to read3P"
                  n82 = Byte Array To String(unsigned byte array=w704) -> (string=w703:string)
                  n83 = String Subset(string=w703, offset (0)=0, length (rest)=w706) -> (substring=w705:string)
                  n84 = Fract/Exp String To Number(string=w705) -> (number=w701:dbl)  [unwired: 3 in, 1 out]
                  n85 = Multiply(x=w701, y="Servo 2 Position Slope") -> (x*y=w702:dbl)
                  n86 = Add(x=w702, y="Servo 2 Position Intercept") -> (x+y=w700:dbl)
                  "Pos2 number" <- w700
                }
              }
            }
            frame "read3P" {
              n87 = Equal?(x=w733, y="d") -> (x = y?=w747:bool)
              n88 = case shown="True" w747 {
                tunnel: [w756 0] -> w737
                tunnel: w746 -> [w750 w763]
                tunnel: w743 -> [w754 w764]
                tunnel: [w753 w764] -> w742
                tunnel: w733 -> [w752 _]
                tunnel: [w749 24] -> w740
                tunnel: w725 -> [w749 _]
                tunnel: [w748 w757] -> w731
                tunnel: w730 -> [w748 _]
                frame False {
                  n89 = String To Byte Array(string=w752) -> (unsigned byte array=w751:u8[])
                  n90 = Insert Into Array(array=w754, index=w750, new element=w751) -> (w753:dbl[])
                  n91 = Add(x=w750, y=1) -> (x+y=w756:i32)
                }
                frame True {
                  # "Go to read4P"
                  n92 = Byte Array To String(unsigned byte array=w764) -> (string=w765:string)
                  n93 = String Subset(string=w765, offset (0)=0, length (rest)=w763) -> (substring=w762:string)
                  n94 = Fract/Exp String To Number(string=w762) -> (number=w760:dbl)  [unwired: 3 in, 1 out]
                  n95 = Multiply(x=w760, y="Servo 3 Position Slope") -> (x*y=w761:dbl)
                  n96 = Add(x=w761, y="Servo 3 Position Intercept") -> (x+y=w757:dbl)
                  "Pos3 number" <- w757
                }
              }
            }
            frame "read4P" {
              n97 = Equal?(x=w800, y="e") -> (x = y?=w802:bool)
              n98 = case shown="True" w802 {
                tunnel: [w815 0] -> w799
                tunnel: w785 -> [w809 w823]
                tunnel: w806 -> [w813 w824]
                tunnel: [w812 w824] -> w805
                tunnel: w800 -> [w811 _]
                tunnel: [w808 30] -> w786
                tunnel: w801 -> [w808 _]
                tunnel: [w807 w820] -> w790
                tunnel: w789 -> [w807 _]
                frame False {
                  n99 = String To Byte Array(string=w811) -> (unsigned byte array=w810:u8[])
                  n100 = Insert Into Array(array=w813, index=w809, new element=w810) -> (w812:dbl[])
                  n101 = Add(x=w809, y=1) -> (x+y=w815:i32)
                }
                frame True {
                  # "Go to read5P"
                  n102 = Byte Array To String(unsigned byte array=w824) -> (string=w825:string)
                  n103 = String Subset(string=w825, offset (0)=0, length (rest)=w823) -> (substring=w822:string)
                  n104 = Fract/Exp String To Number(string=w822) -> (number=w819:dbl)  [unwired: 3 in, 1 out]
                  n105 = Multiply(x=w819, y="Servo 4 Position Slope") -> (x*y=w821:dbl)
                  n106 = Add(x=w821, y="Servo 4 Position Intercept") -> (x+y=w820:dbl)
                  "Pos4 number" <- w820
                }
              }
            }
            frame "read5P" {
              n107 = Equal?(x=w859, y="v") -> (x = y?=w860:bool)
              n108 = case shown="True" w860 {
                tunnel: [w874 0] -> w857
                tunnel: w858 -> [w868 w881]
                tunnel: w864 -> [w872 w882]
                tunnel: [w871 w882] -> w863
                tunnel: w859 -> [w870 _]
                tunnel: [w867 36] -> w862
                tunnel: w861 -> [w867 _]
                tunnel: [w866 w876] -> w847
                tunnel: w845 -> [w866 _]
                frame False {
                  n109 = String To Byte Array(string=w870) -> (unsigned byte array=w869:u8[])
                  n110 = Insert Into Array(array=w872, index=w868, new element=w869) -> (w871:dbl[])
                  n111 = Add(x=w868, y=1) -> (x+y=w874:i32)
                }
                frame True {
                  # "Go to read1T"
                  n112 = Byte Array To String(unsigned byte array=w882) -> (string=w883:string)
                  n113 = String Subset(string=w883, offset (0)=0, length (rest)=w881) -> (substring=w880:string)
                  n114 = Fract/Exp String To Number(string=w880) -> (number=w878:dbl)  [unwired: 3 in, 1 out]
                  n115 = Multiply(x=w878, y="Servo 5 Position Slope") -> (x*y=w879:dbl)
                  n116 = Add(x=w879, y="Servo 5 Position Intercept") -> (x+y=w876:dbl)
                  "Pos5 number" <- w876
                }
              }
            }
            frame "read1T" {
              n117 = Equal?(x=w920, y="w") -> (x = y?=w921:bool)
              n118 = case shown="True" w921 {
                tunnel: [w933 0] -> w902
                tunnel: w903 -> [w927 w939]
                tunnel: w906 -> [w931 w941]
                tunnel: [w930 w941] -> w905
                tunnel: w920 -> [w929 _]
                tunnel: [w926 42] -> w923
                tunnel: w922 -> [w926 _]
                tunnel: [w925 w936] -> w899
                tunnel: w901 -> [w925 _]
                frame False {
                  n119 = String To Byte Array(string=w929) -> (unsigned byte array=w928:u8[])
                  n120 = Insert Into Array(array=w931, index=w927, new element=w928) -> (w930:dbl[])
                  n121 = Add(x=w927, y=1) -> (x+y=w933:i32)
                }
                frame True {
                  # "Go to read2T"
                  n122 = Byte Array To String(unsigned byte array=w941) -> (string=w942:string)
                  n123 = String Subset(string=w942, offset (0)=0, length (rest)=w939) -> (substring=w940:string)
                  n124 = Fract/Exp String To Number(string=w940) -> (number=w937:dbl)  [unwired: 3 in, 1 out]
                  n125 = Multiply(x=w937, y="Servo 1 Torque Slope") -> (x*y=w938:dbl)
                  n126 = Add(x=w938, y="Servo 1 Torque Intercept") -> (x+y=w936:dbl)
                  "Torq1 number" <- w936
                }
              }
            }
            frame "read2T" {
              n127 = Equal?(x=w979, y="x") -> (x = y?=w980:bool)
              n128 = case shown="True" w980 {
                tunnel: [w992 0] -> w954
                tunnel: w953 -> [w986 w998]
                tunnel: w965 -> [w990 w1000]
                tunnel: [w989 w1000] -> w964
                tunnel: w979 -> [w988 _]
                tunnel: [w985 48] -> w982
                tunnel: w981 -> [w985 _]
                tunnel: [w984 w995] -> w949
                tunnel: w952 -> [w984 _]
                frame False {
                  n129 = String To Byte Array(string=w988) -> (unsigned byte array=w987:u8[])
                  n130 = Insert Into Array(array=w990, index=w986, new element=w987) -> (w989:dbl[])
                  n131 = Add(x=w986, y=1) -> (x+y=w992:i32)
                }
                frame True {
                  # "Go to read3T"
                  n132 = Byte Array To String(unsigned byte array=w1000) -> (string=w1001:string)
                  n133 = String Subset(string=w1001, offset (0)=0, length (rest)=w998) -> (substring=w999:string)
                  n134 = Fract/Exp String To Number(string=w999) -> (number=w996:dbl)  [unwired: 3 in, 1 out]
                  n135 = Multiply(x=w996, y="Servo 2 Torque Slope") -> (x*y=w997:dbl)
                  n136 = Add(x=w997, y="Servo 2 Torque Intercept") -> (x+y=w995:dbl)
                  "Torq2 number" <- w995
                }
              }
            }
            frame "read3T" {
              n137 = Equal?(x=w1038, y="y") -> (x = y?=w1039:bool)
              n138 = case shown="True" w1039 {
                tunnel: [w1051 0] -> w1014
                tunnel: w1013 -> [w1045 w1057]
                tunnel: w1017 -> [w1049 w1059]
                tunnel: [w1048 w1059] -> w1016
                tunnel: w1038 -> [w1047 _]
                tunnel: [w1044 54] -> w1041
                tunnel: w1040 -> [w1044 _]
                tunnel: [w1043 w1055] -> w1020
                tunnel: w1025 -> [w1043 _]
                frame False {
                  n139 = String To Byte Array(string=w1047) -> (unsigned byte array=w1046:u8[])
                  n140 = Insert Into Array(array=w1049, index=w1045, new element=w1046) -> (w1048:dbl[])
                  n141 = Add(x=w1045, y=1) -> (x+y=w1051:i32)
                }
                frame True {
                  # "Go to read4T"
                  n142 = Byte Array To String(unsigned byte array=w1059) -> (string=w1060:string)
                  n143 = String Subset(string=w1060, offset (0)=0, length (rest)=w1057) -> (substring=w1058:string)
                  n144 = Fract/Exp String To Number(string=w1058) -> (number=w1054:dbl)  [unwired: 3 in, 1 out]
                  n145 = Multiply(x=w1054, y="Servo 3 Torque Slope") -> (x*y=w1056:dbl)
                  n146 = Add(x=w1056, y="Servo 3 Torque Intercept") -> (x+y=w1055:dbl)
                  "Torq3 number" <- w1055
                }
              }
            }
            frame "read4T" {
              n147 = Equal?(x=w1097, y="z") -> (x = y?=w1098:bool)
              n148 = case shown="True" w1098 {
                tunnel: [w1110 0] -> w1070
                tunnel: w1069 -> [w1104 w1116]
                tunnel: w1075 -> [w1108 w1118]
                tunnel: [w1107 w1118] -> w1076
                tunnel: w1097 -> [w1106 _]
                tunnel: [w1103 60] -> w1100
                tunnel: w1099 -> [w1103 _]
                tunnel: [w1102 w1113] -> w1079
                tunnel: w1083 -> [w1102 _]
                frame False {
                  n149 = String To Byte Array(string=w1106) -> (unsigned byte array=w1105:u8[])
                  n150 = Insert Into Array(array=w1108, index=w1104, new element=w1105) -> (w1107:dbl[])
                  n151 = Add(x=w1104, y=1) -> (x+y=w1110:i32)
                }
                frame True {
                  # "Go to read5T"
                  n152 = Byte Array To String(unsigned byte array=w1118) -> (string=w1119:string)
                  n153 = String Subset(string=w1119, offset (0)=0, length (rest)=w1116) -> (substring=w1117:string)
                  n154 = Fract/Exp String To Number(string=w1117) -> (number=w1114:dbl)  [unwired: 3 in, 1 out]
                  n155 = Multiply(x=w1114, y="Servo 4 Torque Slope") -> (x*y=w1115:dbl)
                  n156 = Add(x=w1115, y="Servo 4 Torque Intercept") -> (x+y=w1113:dbl)
                  "Torq4 number" <- w1113
                }
              }
            }
            frame "read5T" {
              n157 = Equal?(x=w1156, y="!") -> (x = y?=w1157:bool)
              n158 = case shown="True" w1157 {
                tunnel: [w1169 0] -> w1132
                tunnel: w1131 -> [w1163 w1175]
                tunnel: w1134 -> [w1167 w1177]
                tunnel: [w1166 w1177] -> w1135
                tunnel: w1156 -> [w1165 _]
                tunnel: [w1162 0] -> w1159
                tunnel: w1158 -> [w1162 _]
                tunnel: [w1161 w1170] -> w1141
                tunnel: w1142 -> [w1161 _]
                frame False {
                  n159 = String To Byte Array(string=w1165) -> (unsigned byte array=w1164:u8[])
                  n160 = Insert Into Array(array=w1167, index=w1163, new element=w1164) -> (w1166:dbl[])
                  n161 = Add(x=w1163, y=1) -> (x+y=w1169:i32)
                }
                frame True {
                  # "Go to none11"
                  n162 = Byte Array To String(unsigned byte array=w1177) -> (string=w1178:string)
                  n163 = String Subset(string=w1178, offset (0)=0, length (rest)=w1175) -> (substring=w1176:string)
                  n164 = Fract/Exp String To Number(string=w1176) -> (number=w1173:dbl)  [unwired: 3 in, 1 out]
                  n165 = Multiply(x=w1173, y="Servo 5 Torque Slope") -> (x*y=w1174:dbl)
                  n166 = Add(x=w1174, y="Servo 5 Torque Intercept") -> (x+y=w1170:dbl)
                  "Torq5 number" <- w1170
                }
              }
            }
          }
        }
      }
    }
    n167 = Split Signals(w59) -> (w58:dynamicdata, w57:dynamicdata, w56:dynamicdata)  [unwired: 3 in]
    n168 = call "Convert from Dynamic Data3"("Dynamic Data Type"=w58) -> ("Array"=w49:dbl[])  [unwired: 3 in]
    n169 = call "Convert from Dynamic Data"("Dynamic Data Type"=w56) -> ("Array"=w46:dbl[])  [unwired: 3 in]
    n170 = call "Convert from Dynamic Data2"("Dynamic Data Type"=w57) -> ("Array"=w47:dbl[])  [unwired: 3 in]
    n171 = Subtract(x=w80, y=1) -> (x-y=w276:i32)
    n172 = Subtract(x=w80, y=1) -> (x-y=w265:i32)
    n173 = Subtract(x=w80, y=1) -> (x-y=w268:i32)
    n174 = Subtract(x=w80, y=1) -> (x-y=w259:i32)
    n175 = Subtract(x=w80, y=1) -> (x-y=w262:i32)
    n176 = Index Array(array=w263, index=w265) -> (element=w247:dbl)
    n177 = Index Array(array=w266, index=w268) -> (element=w252:dbl)
    n178 = Index Array(array=w260, index=w262) -> (element=w241:dbl)
    n179 = Index Array(array=w230, index=w259) -> (element=w232:dbl)
    n180 = Index Array(array=w274, index=w276) -> (element=w271:dbl)
    n181 = Multiply(x="Drag Force Slope", y=w49) -> (x*y=w55:dbl[])
    n182 = Multiply(x="Lift Force Slope", y=w47) -> (x*y=w52:dbl[])
    n183 = Multiply(x="Yaw Moment Slope", y=w46) -> (x*y=w51:dbl[])
    n184 = Add(x=w52, y="Lift Force Intercept") -> (x+y=w41:dbl[])
    n185 = Less?(x=w235, y="Lowest Servo Angle") -> (x < y?=w236:bool)
    n186 = Greater?(x=w235, y="Highest Servo Angle") -> (0:w238:bool)
    n187 = Add(x=w51, y="Yaw Moment Intercept") -> (x+y=w42:dbl[])
    n188 = Add(x=w55, y="Drag Force Intercept") -> (x+y=w40:dbl[])
    n189 = Or(x=w238, y=w236) -> (x .or. y?=w237:bool)
    n190 = case shown="True" w237 {
      tunnel: w232 -> [_ w421]
      tunnel: w235 -> [w419 _]
      tunnel: [w419 w421] -> w231
      tunnel: [FALSE TRUE] -> w168
      frame False {
      }
      frame True {
      }
    }
    n191 = Greater?(x=w239, y="Highest Servo Angle") -> (0:w242:bool)
    n192 = Less?(x=w239, y="Lowest Servo Angle") -> (x < y?=w243:bool)
    n193 = Or(x=w242, y=w243) -> (x .or. y?=w244:bool)
    n194 = case shown="True" w244 {
      tunnel: w241 -> [_ w425]
      tunnel: w239 -> [w423 _]
      tunnel: [w423 w425] -> w240
      tunnel: [FALSE TRUE] -> w169
      frame False {
      }
      frame True {
      }
    }
    n195 = Or(x=w169, y=w168) -> (x .or. y?=w166:bool)
    n196 = Greater?(x=w245, y="Highest Servo Angle") -> (0:w250:bool)
    n197 = Less?(x=w245, y="Lowest Servo Angle") -> (x < y?=w248:bool)
    n198 = Or(x=w250, y=w248) -> (x .or. y?=w249:bool)
    n199 = case shown="True" w249 {
      tunnel: w247 -> [_ w429]
      tunnel: w245 -> [w427 _]
      tunnel: [w427 w429] -> w246
      tunnel: [FALSE TRUE] -> w167
      frame False {
      }
      frame True {
      }
    }
    n200 = Or(x=w167, y=w166) -> (x .or. y?=w164:bool)
    n201 = Greater?(x=w251, y="Highest Servo Angle") -> (0:w256:bool)
    n202 = Less?(x=w251, y="Lowest Servo Angle") -> (x < y?=w254:bool)
    n203 = Or(x=w256, y=w254) -> (x .or. y?=w255:bool)
    n204 = case shown="True" w255 {
      tunnel: w252 -> [_ w433]
      tunnel: w251 -> [w431 _]
      tunnel: [w431 w433] -> w253
      tunnel: [FALSE TRUE] -> w165
      frame False {
      }
      frame True {
      }
    }
    n205 = Or(x=w165, y=w164) -> (x .or. y?=w162:bool)
    n206 = Less?(x=w269, y="Lowest Servo Angle") -> (x < y?=w270:bool)
    n207 = Greater?(x=w269, y="Highest Servo Angle") -> (0:w273:bool)
    n208 = Or(x=w273, y=w270) -> (x .or. y?=w272:bool)
    n209 = Insert Into Array(array=w78, index=w80, new element=w41) -> (w76:dbl[])
    n210 = Insert Into Array(array=w77, index=w80, new element=w42) -> (w75:dbl[])
    n211 = Insert Into Array(array=w79, index=w80, new element=w40) -> (w74:dbl[])
    n212 = case shown="True" w272 {
      tunnel: w271 -> [_ w437]
      tunnel: w269 -> [w435 _]
      tunnel: [w435 w437] -> w257
      tunnel: [FALSE TRUE] -> w163
      frame False {
      }
      frame True {
      }
    }
    n213 = Or(x=w163, y=w162) -> (x .or. y?=→"Minimum or Maximum Angle Exceeded":bool)
    n214 = call <vilib>:"Amplitude and Phase Spectrum.vi"("dt"=w39, "Signal (V)"=w74) -> ("df"=w70:dbl, "Amp Spectrum Mag (Vrms)"=w71:dbl[])  [unwired: 1 in, 1 out]
    n215 = Insert Into Array(array=w274, index=w80, new element=w257) -> (w147:dbl[])
    n216 = Insert Into Array(array=w266, index=w80, new element=w253) -> (w309:dbl[])
    n217 = Insert Into Array(array=w230, index=w80, new element=w231) -> (w300:dbl[])
    n218 = Insert Into Array(array=w263, index=w80, new element=w246) -> (w306:dbl[])
    n219 = Insert Into Array(array=w260, index=w80, new element=w240) -> (w303:dbl[])
    n220 = Greater?(x=w145, y="Max Torque") -> (0:w139:bool)
    n221 = Bundle("timeout (s)"=0.0, "df"=w70, "Amp Spectrum Mag (Vrms)"=w71) -> (→"Lift FFT":T3)  [unwired: 1 in]
    n222 = Greater?(x=w141, y="Max Torque") -> (0:w138:bool)
    n223 = Greater?(x=w142, y="Max Torque") -> (0:w137:bool)
    n224 = Or(x=w138, y=w139) -> (x .or. y?=w136:bool)
    n225 = Greater?(x=w143, y="Max Torque") -> (0:w135:bool)
    n226 = Or(x=w137, y=w136) -> (x .or. y?=w132:bool)
    n227 = Greater?(x=w144, y="Max Torque") -> (0:w134:bool)
    n228 = Or(x=w135, y=w132) -> (x .or. y?=w133:bool)
    n229 = Bundle(w65, 20, 0.5, 0.1, w65) -> (w69:cluster{i32, i32, dbl, dbl, i32})  [unwired: 1 in]
    n230 = Subtract(x=w113, y=w117) -> (x-y=w118:dbl)
    n231 = Bundle(w61, 1, 0.1, 0.05, w61) -> (w60:cluster{i32, i32, dbl, dbl, i32})  [unwired: 1 in]
    n232 = Insert Into Array(array=w285, index=w80, new element=w145) -> (w160:dbl[])
    n233 = Insert Into Array(array=w284, index=w80, new element=w141) -> (w158:dbl[])
    n234 = Insert Into Array(array=w281, index=w80, new element=w144) -> (w159:dbl[])
    n235 = Or(x=w134, y=w133) -> (x .or. y?=→"Maximum Torque Exceeded":bool)
    n236 = Insert Into Array(array=w283, index=w80, new element=w142) -> (w157:dbl[])
    n237 = Subtract(x=w114, y=w117) -> (x-y=w119:dbl)
    n238 = Insert Into Array(array=w282, index=w80, new element=w143) -> (w156:dbl[])
    n239 = Subtract(x=w112, y=w117) -> (x-y=w120:dbl)
    n240 = property on="Lift FFT" class="WFGraph (strict)"("XScale.Range"=w69) -> ()  [unwired: 2 in, 2 out]
    n241 = Subtract(x=w115, y=w117) -> (x-y=w121:dbl)
    n242 = Subtract(x=w116, y=w117) -> (x-y=w122:dbl)
    n243 = property on="Lift FFT" class="WFGraph (strict)"("YScale.Range"=w60) -> ()  [unwired: 2 in, 2 out]
    n244 = Build Array(w122, w121, w120, w119, w118) -> (w86:dbl[])
    "Output Angles" <- w86
    n245 = Build Array(w147, w313) -> (w312:dbl[][])
    n246 = Build Array(w309, w310) -> (w311:dbl[][])
    n247 = Build Array(w306, w307) -> (w308:dbl[][])
    n248 = Build Array(w303, w304) -> (w305:dbl[][])
    n249 = Build Array(w300, w301) -> (w302:dbl[][])
    n250 = Bundle(0, w39, w311) -> (→"Servo 2 Position":cluster{i32, dbl, dbl[][]})  [unwired: 1 in]
    n251 = Bundle(0, w39, w302) -> (→"Servo 5 Position":cluster{i32, dbl, dbl[][]})  [unwired: 1 in]
    n252 = Divide(x="Length of Segments", y=100) -> (x/y=w98:dbl)
    n253 = Bundle(0, w39, w312) -> (→"Servo 1 Position":cluster{i32, dbl, dbl[][]})  [unwired: 1 in]
    n254 = Initialize Array(0.0 ("element"), 1 ("dimension size")) -> (w125:dbl[])
    n255 = Bundle(0, w39, w305) -> (→"Servo 4 Position":cluster{i32, dbl, dbl[][]})  [unwired: 1 in]
    n256 = Bundle(0, w39, w308) -> (→"Servo 3 Position":cluster{i32, dbl, dbl[][]})  [unwired: 1 in]
    n257 = Initialize Array(0.0 ("element"), 1 ("dimension size")) -> (w124:dbl[])
    n258 = call "PlotSubArray.vi"("Time Step (s)"=w39, "Plot Last x Seconds"="Plot Last x Seconds", "Iteration"=w80, "Array"=w160) -> ("Sub Array"=w154:dbl[], "Time Offset"=w155:dbl)  [unwired: 6 in]
    n259 = call "PlotSubArray.vi"("Time Step (s)"=w39, "Plot Last x Seconds"="Plot Last x Seconds", "Iteration"=w80, "Array"=w158) -> ("Sub Array"=w153:dbl[])  [unwired: 6 in, 1 out]
    n260 = call "PlotSubArray.vi"("Time Step (s)"=w39, "Plot Last x Seconds"="Plot Last x Seconds", "Iteration"=w80, "Array"=w157) -> ("Sub Array"=w152:dbl[])  [unwired: 6 in, 1 out]
    n261 = call "PlotSubArray.vi"("Time Step (s)"=w39, "Plot Last x Seconds"="Plot Last x Seconds", "Iteration"=w80, "Array"=w156) -> ("Sub Array"=w151:dbl[])  [unwired: 6 in, 1 out]
    n262 = call "PlotSubArray.vi"("Time Step (s)"=w39, "Plot Last x Seconds"="Plot Last x Seconds", "Iteration"=w80, "Array"=w159) -> ("Sub Array"=w150:dbl[])  [unwired: 6 in, 1 out]
    n263 = Build Array(w154, w153, w152, w151, w150) -> (w149:dbl[][])
    n264 = for {
      N: "Number of Servos" -> [_]
      shift-right: [w363] -> _
      shift-left: 0.0 -> [w380]
      tunnel: w86 -> [w379]
      shift-right: [w373] -> w94
      shift-left: w125 -> [w361]
      shift-right: [w372] -> w93
      shift-left: w124 -> [w360]
      tunnel: w98 -> [w359]
      i -> [w371]
      (unwired) 100
      # "phi"
      # "L"
      n265 = Index Array(array=w379, index=w371) -> (element=w378:dbl)
      n266 = Index Array(array=w361, index=w371) -> (element=w377:dbl)
      n267 = Index Array(array=w360, index=w371) -> (element=w374:dbl)
      n268 = Divide(x=3.141592653589793, y=180) -> (x/y=w362:dbl)
      n269 = Add(x=w378, y=w380) -> (x+y=w363:dbl)
      n270 = Multiply(x=w362, y=w363) -> (x*y=w365:dbl)
      n271 = Multiply(x=w362, y=w363) -> (x*y=w364:dbl)
      n272 = Increment(x=w371) -> (x+1=w370:i32)
      n273 = Cosine(x=w365) -> (cos(x)=w369:dbl)
      n274 = Sine(x=w364) -> (sin(x)=w368:dbl)
      n275 = Multiply(x=w369, y=w359) -> (x*y=w376:dbl)
      n276 = Multiply(x=w359, y=w368) -> (x*y=w375:dbl)
      n277 = Add(x=w377, y=w376) -> (x+y=w358:dbl)
      n278 = Add(x=w375, y=w374) -> (x+y=w357:dbl)
      n279 = Insert Into Array(array=w361, index=w370, new element=w358) -> (w373:dbl[])
      n280 = Insert Into Array(array=w360, index=w370, new element=w357) -> (w372:dbl[])
    }
    n281 = Bundle("Time Offset"=w155, w39, w149) -> (→"Servo Torque":cluster{" Time Offset":dbl, dbl, dbl[][]})  [unwired: 1 in]
    n282 = Increment(x="Number of Servos") -> (x+1=w111:dbl)
    n283 = Increment(x="Number of Servos") -> (x+1=w108:dbl)
    n284 = Increment(x="Number of Servos") -> (x+1=w95:dbl)
    n285 = Build Array(w74, w76, w75) -> (w81:dbl[][])
    n286 = Bundle(0, w39, w81) -> (→"Force and Torque Data":cluster{i32, dbl, dbl[][]})  [unwired: 1 in]
    n287 = Multiply(x=w111, y="Length of Segments") -> (x*y=w109:dbl)
    n288 = Multiply(x=w108, y="Length of Segments") -> (x*y=w105:dbl)
    n289 = Divide(x="Length of Segments", y=5) -> (x/y=w106:dbl)
    n290 = Divide(x="Length of Segments", y=5) -> (x/y=w107:dbl)
    n291 = Multiply(x=-1, y=w109) -> (x*y=w110:dbl)
    n292 = Bundle(w101, w105, w98, w106, w101) -> (w100:cluster{i32, dbl, dbl, dbl, i32})  [unwired: 1 in]
    n293 = for {
      N: w95 -> [_]
      tunnel: w94 -> [w356] mode=indexing
      tunnel: w93 -> [w354] mode=indexing
      tunnel: [w353] -> w90 mode=indexing
      tunnel: [w352] -> w89 mode=indexing
      w355 = 100
      # "Convert nodes from m to cm"
      n294 = Multiply(x=w356, y=w355) -> (x*y=w353:dbl)
      n295 = Multiply(x=w355, y=w354) -> (x*y=w352:dbl)
    }
    n296 = Bundle(w110, w109, w98, w107, w110) -> (w99:cluster{dbl, dbl, dbl, dbl, dbl})  [unwired: 1 in]
    n297 = property on="Waveform" class="XYGraph (strict)"("XScale.Range"=w100) -> ()  [unwired: 2 in, 2 out]
    n298 = property on="Waveform" class="XYGraph (strict)"("YScale.Range"=w99) -> ()  [unwired: 2 in, 2 out]
    n299 = property on="Waveform" class="XYGraph (strict)"("Plot.Point Style"=u8 2) -> ()  [unwired: 2 in, 2 out]
    n300 = Bundle(w90, w89) -> (w88:cluster{dbl[], dbl[]})  [unwired: 1 in]
    n301 = Build Array(w96, w88) -> (→"Waveform":cluster{"X Nodes":dbl[], "Y Nodes":dbl[]}[])
  }
  n302 = VISA Close(VISA resource name=w22, error in (no error)=w21) -> ()  [unwired: 1 out]
  n303 = case shown="True" w23 {
    tunnel: w24 -> [_ w1256]
    tunnel: w20 -> [_ w1255]
    tunnel: w16 -> [_ w1244]
    tunnel: w15 -> [_ w1243]
    tunnel: w14 -> [_ w1242]
    tunnel: w13 -> [_ w1233]
    tunnel: w12 -> [_ w1232]
    tunnel: w11 -> [_ w1231]
    tunnel: w10 -> [_ w1230]
    tunnel: w9 -> [_ w1221]
    tunnel: w8 -> [_ w1220]
    tunnel: w7 -> [_ w1219]
    tunnel: w6 -> [_ w1218]
    tunnel: w5 -> [_ w1216]
    tunnel: w4 -> [_ w1206]
    tunnel: w3 -> [_ w1205]
    tunnel: w2 -> [_ w1204]
    tunnel: w1 -> [_ w1203]
    frame False {
    }
    frame True {
      n304 = call "Convert to Dynamic Data9"("Array"=w1230) -> ("Dynamic Data Type"=w1235:dynamicdata)  [unwired: 3 in]
      n305 = call "Convert to Dynamic Data11"("Array"=w1220) -> ("Dynamic Data Type"=w1227:dynamicdata)  [unwired: 3 in]
      n306 = call "Convert to Dynamic Data13"("Array"=w1218) -> ("Dynamic Data Type"=w1223:dynamicdata)  [unwired: 3 in]
      n307 = call "Convert to Dynamic Data"("Array"=w1255) -> ("Dynamic Data Type"=w1254:dynamicdata)  [unwired: 3 in]
      n308 = call "Convert to Dynamic Data12"("Array"=w1219) -> ("Dynamic Data Type"=w1225:dynamicdata)  [unwired: 3 in]
      n309 = call "Convert to Dynamic Data10"("Array"=w1221) -> ("Dynamic Data Type"=w1229:dynamicdata)  [unwired: 3 in]
      n310 = call "Convert to Dynamic Data17"("Array"=w1204) -> ("Dynamic Data Type"=w1209:dynamicdata)  [unwired: 3 in]
      n311 = call "Convert to Dynamic Data18"("Array"=w1203) -> ("Dynamic Data Type"=w1207:dynamicdata)  [unwired: 3 in]
      n312 = call "Convert to Dynamic Data16"("Array"=w1205) -> ("Dynamic Data Type"=w1211:dynamicdata)  [unwired: 3 in]
      n313 = call "Convert to Dynamic Data15"("Array"=w1206) -> ("Dynamic Data Type"=w1213:dynamicdata)  [unwired: 3 in]
      n314 = call "Convert to Dynamic Data14"("Array"=w1216) -> ("Dynamic Data Type"=w1215:dynamicdata)  [unwired: 3 in]
      n315 = call "Convert to Dynamic Data2"("Array"=w1256) -> ("Dynamic Data Type"=w1253:dynamicdata)  [unwired: 3 in]
      n316 = call "Convert to Dynamic Data6"("Array"=w1233) -> ("Dynamic Data Type"=w1241:dynamicdata)  [unwired: 3 in]
      n317 = call "Convert to Dynamic Data8"("Array"=w1231) -> ("Dynamic Data Type"=w1237:dynamicdata)  [unwired: 3 in]
      n318 = call "Convert to Dynamic Data7"("Array"=w1232) -> ("Dynamic Data Type"=w1239:dynamicdata)  [unwired: 3 in]
      n319 = call "Convert to Dynamic Data5"("Array"=w1244) -> ("Dynamic Data Type"=w1249:dynamicdata)  [unwired: 3 in]
      n320 = call "Convert to Dynamic Data4"("Array"=w1243) -> ("Dynamic Data Type"=w1248:dynamicdata)  [unwired: 3 in]
      n321 = call "Convert to Dynamic Data3"("Array"=w1242) -> ("Dynamic Data Type"=w1250:dynamicdata)  [unwired: 3 in]
      n322 = xnode "Set Dynamic Data Attributes"("Signals In"=w1248, "Signal Name"="Lift Force") -> ("Signals Out"=w1201:dynamicdata)  [unwired: 2 in, 1 out]
      n323 = xnode "Set Dynamic Data Attributes"("Signals In"=w1249, "Signal Name"="Drag Force") -> ("Signals Out"=w1202:dynamicdata)  [unwired: 2 in, 1 out]
      n324 = xnode "Set Dynamic Data Attributes"("Signals In"=w1250, "Signal Name"="Yaw Moment") -> ("Signals Out"=w1200:dynamicdata)  [unwired: 2 in, 1 out]
      n325 = xnode "Set Dynamic Data Attributes"("Signals In"=w1253, "Signal Name"="Servo 1 Commanded Position") -> ("Signals Out"=w1199:dynamicdata)  [unwired: 2 in, 1 out]
      n326 = xnode "Set Dynamic Data Attributes"("Signals In"=w1241, "Signal Name"="Servo 2 Commanded Position") -> ("Signals Out"=w1198:dynamicdata)  [unwired: 2 in, 1 out]
      n327 = xnode "Set Dynamic Data Attributes"("Signals In"=w1237, "Signal Name"="Servo 4 Commanded Position") -> ("Signals Out"=w1196:dynamicdata)  [unwired: 2 in, 1 out]
      n328 = xnode "Set Dynamic Data Attributes"("Signals In"=w1239, "Signal Name"="Servo 3 Commanded Position") -> ("Signals Out"=w1197:dynamicdata)  [unwired: 2 in, 1 out]
      n329 = xnode "Set Dynamic Data Attributes"("Signals In"=w1235, "Signal Name"="Servo 5 Commanded Position") -> ("Signals Out"=w1195:dynamicdata)  [unwired: 2 in, 1 out]
      n330 = xnode "Set Dynamic Data Attributes"("Signals In"=w1254, "Signal Name"="Servo 1 Feedback Position") -> ("Signals Out"=w1194:dynamicdata)  [unwired: 2 in, 1 out]
      n331 = xnode "Set Dynamic Data Attributes"("Signals In"=w1225, "Signal Name"="Servo 1 Feedback Position") -> ("Signals Out"=w1191:dynamicdata)  [unwired: 2 in, 1 out]
      n332 = xnode "Set Dynamic Data Attributes"("Signals In"=w1227, "Signal Name"="Servo 1 Feedback Position") -> ("Signals Out"=w1192:dynamicdata)  [unwired: 2 in, 1 out]
      n333 = xnode "Set Dynamic Data Attributes"("Signals In"=w1209, "Signal Name"="Servo 4  Torque") -> ("Signals Out"=w1186:dynamicdata)  [unwired: 2 in, 1 out]
      n334 = xnode "Set Dynamic Data Attributes"("Signals In"=w1207, "Signal Name"="Servo 5  Torque") -> ("Signals Out"=w1185:dynamicdata)  [unwired: 2 in, 1 out]
      n335 = xnode "Set Dynamic Data Attributes"("Signals In"=w1229, "Signal Name"="Servo 1 Feedback Position") -> ("Signals Out"=w1193:dynamicdata)  [unwired: 2 in, 1 out]
      n336 = xnode "Set Dynamic Data Attributes"("Signals In"=w1211, "Signal Name"="Servo 3  Torque") -> ("Signals Out"=w1187:dynamicdata)  [unwired: 2 in, 1 out]
      n337 = xnode "Set Dynamic Data Attributes"("Signals In"=w1223, "Signal Name"="Servo 1 Feedback Position") -> ("Signals Out"=w1190:dynamicdata)  [unwired: 2 in, 1 out]
      n338 = xnode "Set Dynamic Data Attributes"("Signals In"=w1213, "Signal Name"="Servo 2  Torque") -> ("Signals Out"=w1188:dynamicdata)  [unwired: 2 in, 1 out]
      n339 = xnode "Set Dynamic Data Attributes"("Signals In"=w1215, "Signal Name"="Servo 1  Torque") -> ("Signals Out"=w1189:dynamicdata)  [unwired: 2 in, 1 out]
      n340 = Merge Signals(w1202, w1201, w1200, w1199, w1198, w1197, w1196, w1195, w1194, w1193, w1192, w1191, w1190, w1189, w1188, w1187, w1186, w1185) -> (w1184:dynamicdata)
      n341 = call "Write To Measurement File"("Signals"=w1184, "Filename"="Filename", "Comment"="Comment") -> ()  [unwired: 14 in, 3 out]
    }
  }
